vi "Main.vi"(8 "error in":errorcluster, 11 "Head Worker in":refnum<class "Head Worker.lvclass">) -> (0 "error out":errorcluster, 3 "Head Worker out":refnum<class "Head Worker.lvclass">)   [LabVIEW 2017, in "Method 2.lvlib" / "Head Worker.lvclass"]
doc: "The <b>Queued Message Handler</b> of the Worker that owns this VI."
uses:
  Head Worker.lvclass
  C:/Program Files (x86)/National Instruments/LabVIEW 2017/vi.lib/addons/_Workers/Library/Classes/Worker/Worker.lvclass
  Head Worker.lvclass/Head Worker.ctl
  Initialization Data.ctl
  Response Cases.ctl
  <vilib>/addons/_Workers/Library/Classes/Message Queue/Message Queue.lvclass
  First Level Worker/First Level Worker.lvclass
panel:
  out "subWorker error":errorcluster
  # "Method 2 : Using the Workers Palette \"Send Error to Owner\" VI"
  # "Head Worker (Main VI)"
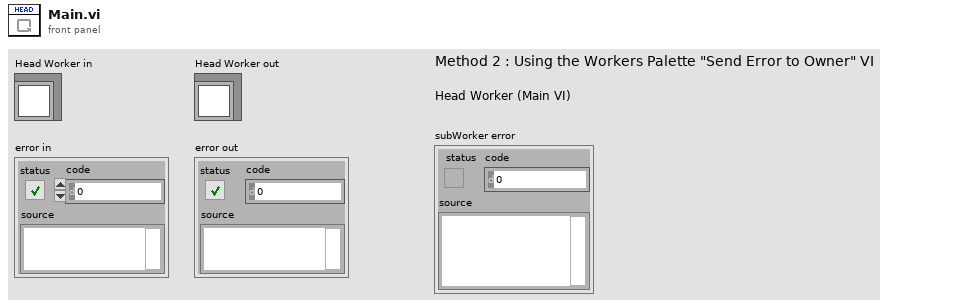
[diagram p1: front panel]
types:
  T1 = typedef "Method 2.lvlib/Head Worker.lvclass/Initialization Data.ctl" = cluster{"Response Cases":T2}
  T2 = typedef "Method 2.lvlib/Head Worker.lvclass/Response Cases.ctl" = cluster{"Placeholder - Can be deleted":string}
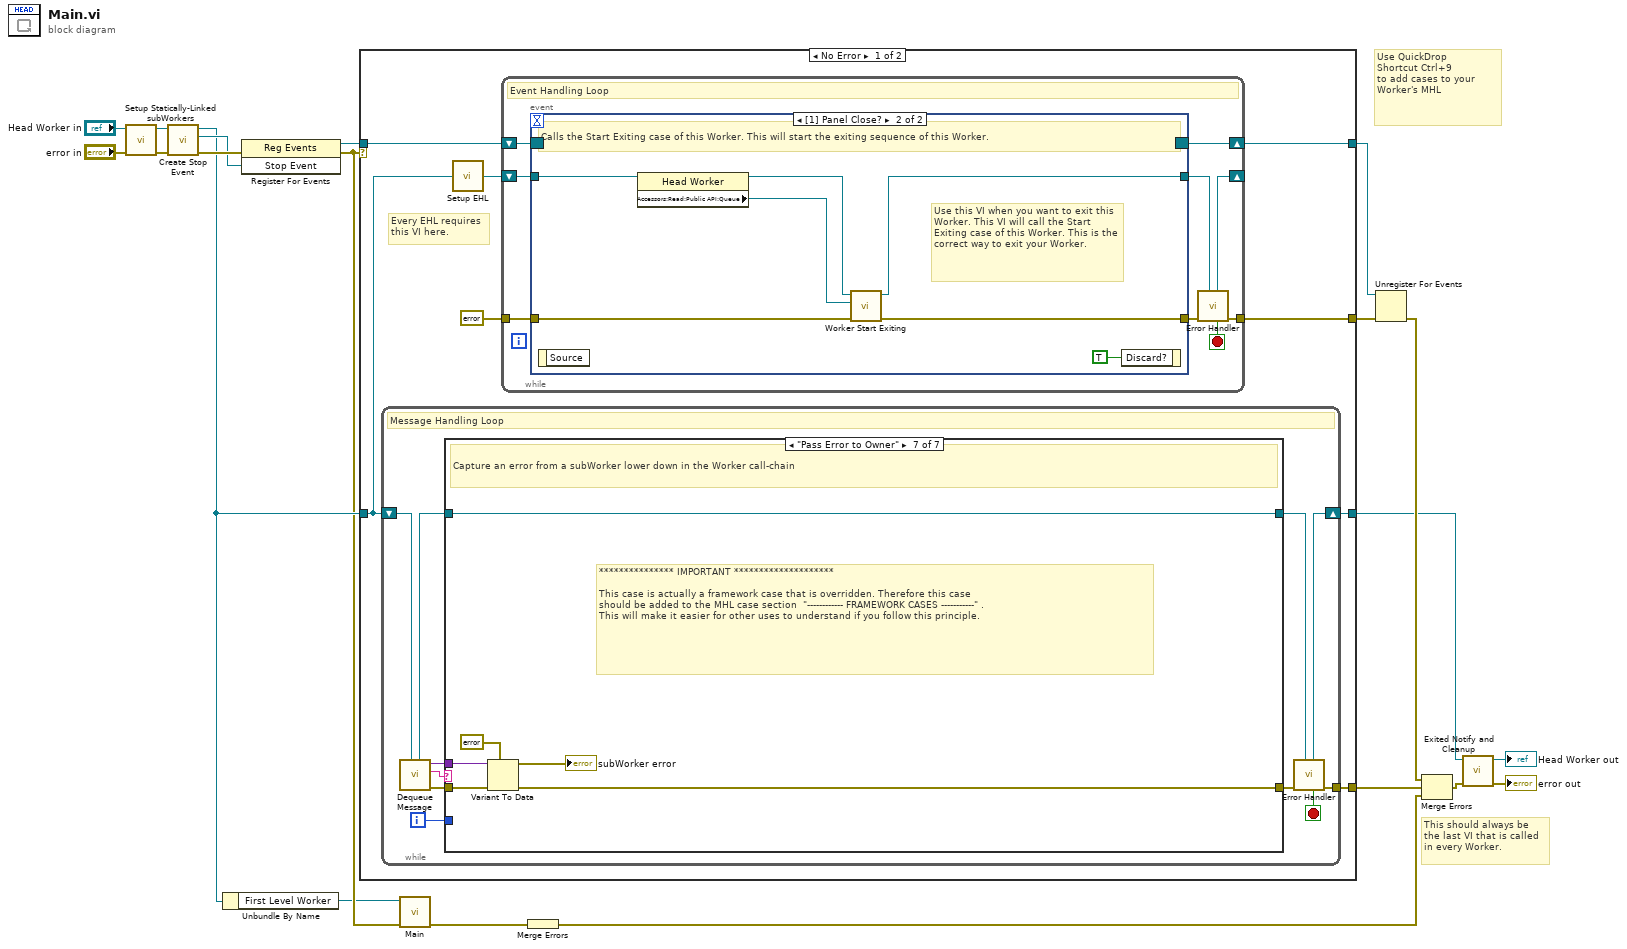
[diagram p0: block diagram]
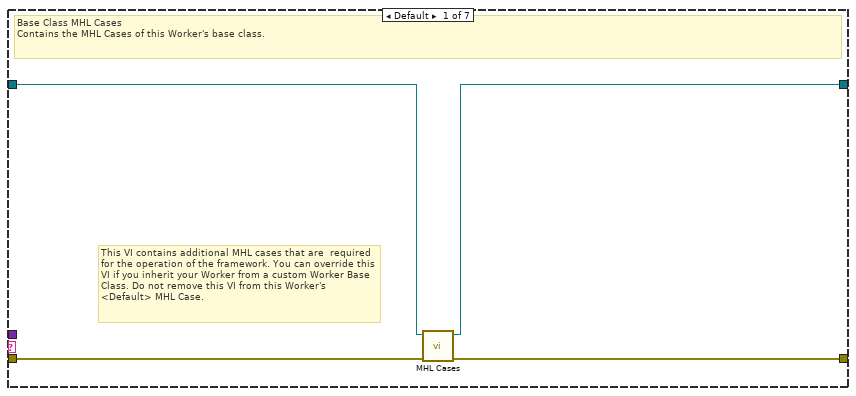
[diagram p2: hidden frame]
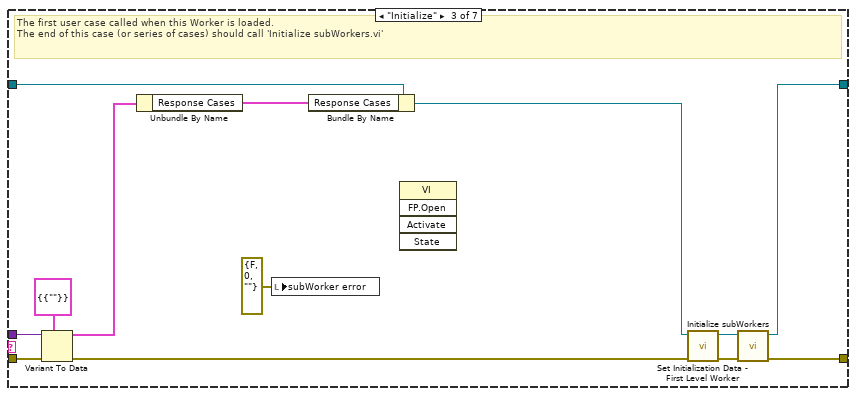
[diagram p4: hidden frame]
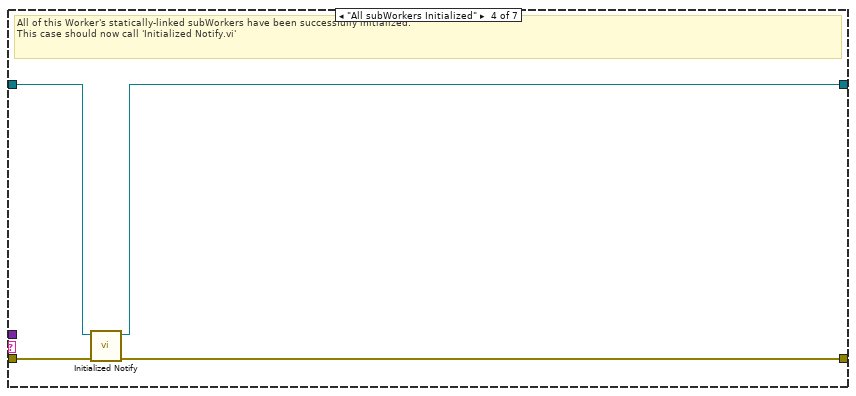
[diagram p5: hidden frame]
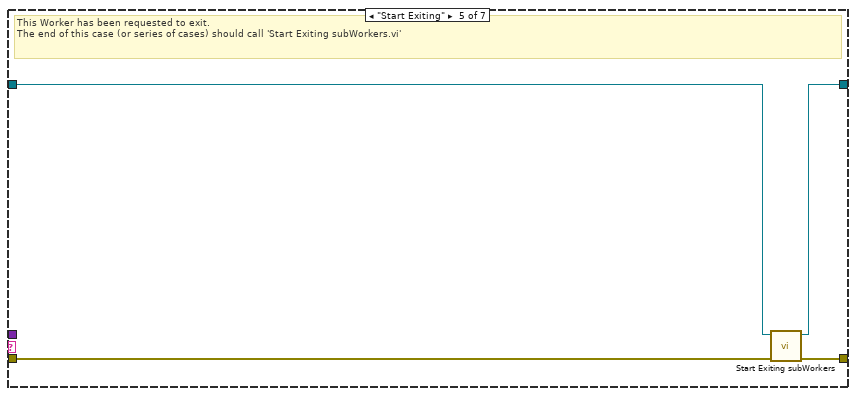
[diagram p6: hidden frame]
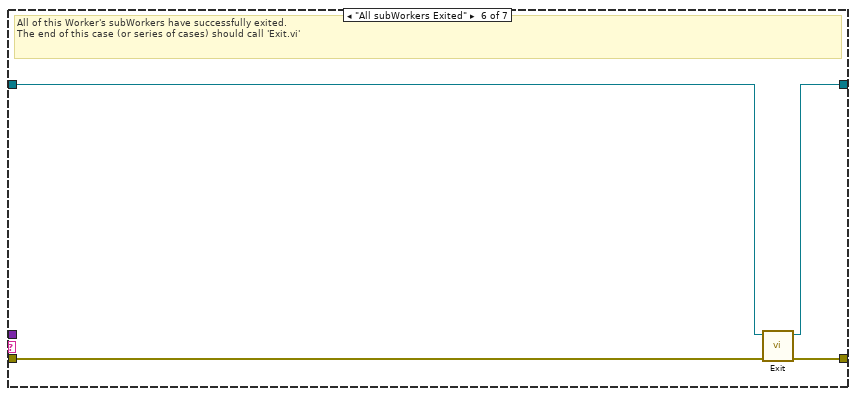
[diagram p7: hidden frame]
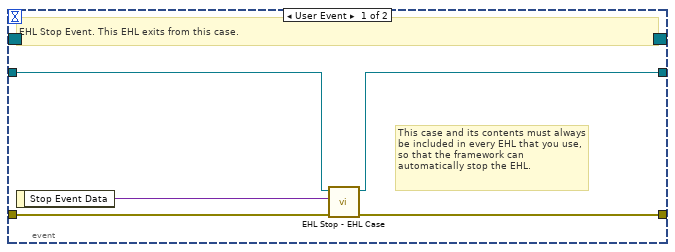
[diagram p8: hidden frame]
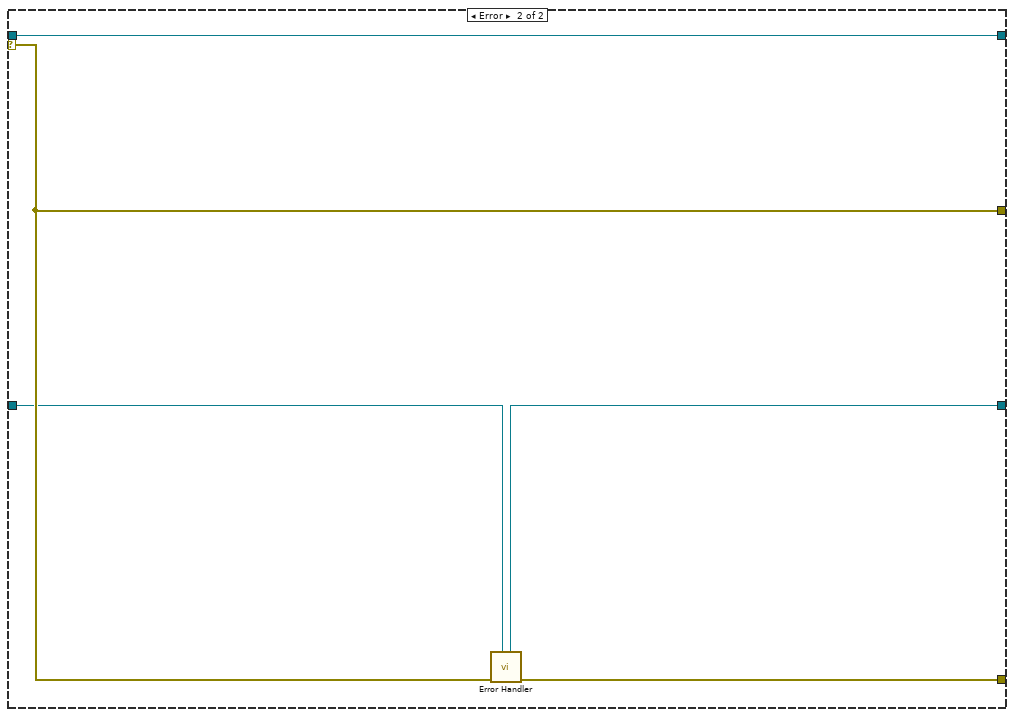
[diagram p9: hidden frame]
diagram:
  # "Use QuickDrop\nShortcut Ctrl+9\nto add cases to your\nWorker's MHL"
  # "This should always be the last VI that is called in every Worker."
  n1 = call "Setup Statically-Linked subWorkers.vi"("error in"="error in", "Head Worker in"="Head Worker in") -> ("error out"=w6:errorcluster, "Head Worker out"=w4:refnum<class "Head Worker.lvclass">)  [unwired: 8 in]
  n2 = call-dynamic "Create Stop Event.vi"("error in"=w6, "Worker"=w4) -> ("error out"=w15:errorcluster, "Stop Event"=w12:refnum<user-event>, "Worker out"=w9:refnum<class "Head Worker.lvclass">)  [unwired: 7 in]
  n3 = Unbundle By Name(w9) -> ("First Level Worker"=w1:refnum<class "First Level Worker.lvclass">)
  n4 = register-events(error in=w15, w12) -> (reference out=w14:refnum<event-registration>, error out=w7:errorcluster)  [unwired: 1 in]
  n5 = case shown="No Error" w7 {
    tunnel: w9 -> [w23 w99]
    tunnel: [w21 w100] -> w13
    tunnel: w14 -> [w28 w101]
    tunnel: [w25 w102] -> w19
    tunnel: [w27 w101] -> w18
    tunnel: [w22 w98] -> w16
    selector: w7 -> [_ w102]
    frame No Error {
      # "Every EHL requires\nthis VI here."
      n6 = while {
        shift-right: [w37] -> w22
        shift-left: w23 -> [w39]
        tunnel: [w38] -> w21
        i -> [w29]
        stop <- w30 stop-if-true
        # "Message Handling Loop"
        n7 = call-dynamic "Dequeue Message.vi"("Worker"=w39) -> ("error out"=w36:errorcluster, "Case out"=w31:string, "Data out"=w32:variant, "Worker out"=w34:refnum<class "Head Worker.lvclass">)  [unwired: 6 in, 1 out]
        n8 = case "Worker MHL Case Structure (DO NOT CHANGE LABEL NAME)" shown="\"Pass Error to Owner\"" w31 {
          tunnel: w36 -> [w43 w44 w56 w60 w63 w70 w76]
          tunnel: [w42 w44 w58 w59 w66 w69 w74] -> w35
          tunnel: w34 -> [w41 w45 w55 w62 w64 w68 w75]
          tunnel: [w40 w45 w57 w61 w65 w67 w75] -> w33
          tunnel: w32 -> [_ _ w53 _ _ _ w73]
          tunnel: w29 -> [_ _ _ _ _ _ _]
          frame Default {
            # "This VI contains additional MHL cases that are  required for the operation of the framework. You can override this VI if you inherit your Worker from a custom Worker Base Class. Do not remove this VI from this Worker's <Default> MHL Case."
            # "Base Class MHL Cases\nContains the MHL Cases of this Worker's base class."
            n9 = call-dynamic "MHL Cases.vi"("error in"=w43, "Worker in"=w41) -> ("error out"=w42:errorcluster, "Worker out"=w40:refnum<class "Head Worker.lvclass">)  [unwired: 8 in]
          }
          frame "------------ FRAMEWORK CASES -----------" {
            # "Start of Workers Framework Cases"
          }
          frame "Initialize" {
            # "The first user case called when this Worker is loaded.\nThe end of this case (or series of cases) should call 'Initialize subWorkers.vi'"
            n10 = Variant To Data(error in=w56, type=T1 {"Response Cases"={"Placeholder - Can be deleted"=""}} ("Initialization Data"), Variant=w53) -> (data=w52:T1, error out=w54:errorcluster)
            n11 = Unbundle By Name(w52) -> ("Response Cases"=w51:T2)
            n12 = local write "subWorker error"(errorcluster {"status"=FALSE, "code"=0, "source"=""} ("subWorker error")) -> ()
            n13 = Bundle By Name(cluster=w55, "Response Cases"=w51) -> (w47:refnum<class "Head Worker.lvclass">)
            n14 = invoke class="VI" method="FP.Open"() -> ()  [unwired: 5 in, 5 out]
            n15 = call "Set Initialization Data - First Level Worker.vi"("error in"=w54, "Head Worker in"=w47) -> ("error out"=w49:errorcluster, "Head Worker out"=w48:refnum<class "Head Worker.lvclass">)  [unwired: 8 in]
            n16 = call-dynamic "Initialize subWorkers.vi"("error in"=w49, "Worker"=w48) -> ("error out"=w58:errorcluster, "dup Worker out"=w57:refnum<class "Head Worker.lvclass">)  [unwired: 8 in]
          }
          frame "All subWorkers Initialized" {
            # "All of this Worker's statically-linked subWorkers have been successfully initialized.\nThis case should now call 'Initialized Notify.vi'"
            n17 = call-dynamic "Initialized Notify.vi"("error in"=w60, "Worker"=w62) -> ("error out"=w59:errorcluster, "dup Worker out"=w61:refnum<class "Head Worker.lvclass">)  [unwired: 8 in]
          }
          frame "Start Exiting" {
            # "This Worker has been requested to exit. \nThe end of this case (or series of cases) should call 'Start Exiting subWorkers.vi'"
            n18 = call-dynamic "Start Exiting subWorkers.vi"("error_in"=w63, "Worker"=w64) -> ("error out"=w66:errorcluster, "dup Worker out"=w65:refnum<class "Head Worker.lvclass">)  [unwired: 8 in]
          }
          frame "All subWorkers Exited" {
            # "All of this Worker's subWorkers have successfully exited. \nThe end of this case (or series of cases) should call 'Exit.vi'"
            n19 = call-dynamic "Exit.vi"("error_in"=w70, "Worker"=w68) -> ("error out"=w69:errorcluster, "dup Worker out"=w67:refnum<class "Head Worker.lvclass">)  [unwired: 8 in]
          }
          frame "Pass Error to Owner" {
            # "*************** IMPORTANT ********************\n\nThis case is actually a framework case that is overridden. Therefore this case\nshould be added to the MHL case section  \"------------ FRAMEWORK CASES -----------\" .\nThis will make it easier for other uses to understand if you follow this principle."
            # "Capture an error from a subWorker lower down in the Worker call-chain"
            n20 = Variant To Data(error in=w76, type=errorcluster {"status"=FALSE, "code"=0, "source"=""} ("error constant"), Variant=w73) -> (data=→"subWorker error":errorcluster, error out=w74:errorcluster)
          }
        }
        n21 = call-dynamic "Error Handler.vi"("Worker"=w33, "error_in"=w35) -> ("error out"=w38:errorcluster, "Stop Loop"=w30:bool, "Worker out"=w37:refnum<class "Head Worker.lvclass">)  [unwired: 7 in]
      }
      n22 = call-dynamic "Setup EHL.vi"("Worker"=w23) -> ("Worker out"=w24:refnum<class "Head Worker.lvclass">)  [unwired: 14 in]
      n23 = while "Event Handling Loop" {
        shift-right: [w85] -> w27
        shift-left: w28 -> [w84]
        tunnel: [w80] -> w25
        tunnel: errorcluster {"status"=FALSE, "code"=0, "source"=""} ("error constant") -> [w82]
        shift-right: [w78] -> _
        shift-left: w24 -> [w83]
        stop <- w77 stop-if-true
        # "Event Handling Loop"
        n24 = event shown="[1] Panel Close?" {
          selector: w84 -> [_ _]
          dyn-events: [_ _] -> w85
          timeout: _ -> [_ _]
          tunnel: [w89 w96] -> w81
          tunnel: w82 -> [w90 w95]
          tunnel: w83 -> [w88 w94]
          tunnel: [w87 w93] -> w79
          event User Event {
            # "This case and its contents must always be included in every EHL that you use, so that the framework can automatically stop the EHL."
            # "EHL Stop Event. This EHL exits from this case."
            n25 = event-data() -> ("Stop Event Data"=w86:variant)  [unwired: 1 in]
            n26 = call-dynamic "EHL Stop - EHL Case.vi"("error in"=w90, "Stop Event Data"=w86, "Worker"=w88) -> ("error out"=w89:errorcluster, "Worker out"=w87:refnum<class "Head Worker.lvclass">)  [unwired: 7 in]
          }
          event Panel Close? {
            # "Use this VI when you want to exit this Worker. This VI will call the Start Exiting case of this Worker. This is the correct way to exit your Worker."
            # "Calls the Start Exiting case of this Worker. This will start the exiting sequence of this Worker."
            n27 = event-data() -> ()  [unwired: 1 in, 1 out]
            n28 = property class="Head Worker"(reference=w94) -> (reference out=w92:refnum<class "Head Worker.lvclass">, "Accessors:Read:Public API:Queue"=w91:refnum<class "Message Queue.lvclass">)  [unwired: 1 in, 1 out]
            n29 = call-dynamic "Worker Start Exiting.vi"("error_in"=w95, "Message Queue"=w91, "Worker"=w92) -> ("error out"=w96:errorcluster, "dup Worker out"=w93:refnum<class "Head Worker.lvclass">)  [unwired: 7 in]
            n30 = event-data ("Event Filter Node")("Discard?"=TRUE) -> ()  [unwired: 1 in, 1 out]
          }
        }
        n31 = call-dynamic "Error Handler.vi"("Worker"=w79, "error_in"=w81) -> ("error out"=w80:errorcluster, "Stop Loop"=w77:bool, "Worker out"=w78:refnum<class "Head Worker.lvclass">)  [unwired: 7 in]
      }
    }
    frame Error {
      n32 = call-dynamic "Error Handler.vi"("Worker"=w99, "error_in"=w102) -> ("error out"=w100:errorcluster, "Worker out"=w98:refnum<class "Head Worker.lvclass">)  [unwired: 7 in, 1 out]
    }
  }
  n33 = call-dynamic "Main.vi"("error in"=w7, "First Level Worker in"=w1) -> ("error out"=w3:errorcluster)  [unwired: 8 in, 1 out]
  n34 = Merge Errors(w3) -> (w2:errorcluster)
  n35 = Unregister For Events(event registration refnum=w18, error in=w19) -> (error out=w20:errorcluster)
  n36 = Merge Errors(w20, w13, w2) -> (w17:errorcluster)
  n37 = call-dynamic "Exited Notify and Cleanup.vi"("error_in"=w17, "Worker"=w16) -> ("error out"=→"error out":errorcluster, "dup Worker out"=→"Head Worker out":refnum<class "Head Worker.lvclass">)  [unwired: 8 in]
